vi "SM - Save settings to non-volatile memory.vi"(1 "error in":errorcluster, 2 "Address / Port":i16=1 min=1 max=31 step=1) -> (0 "error out":errorcluster)   [LabVIEW 2014]
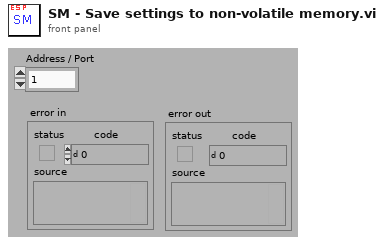
[diagram p1: front panel]
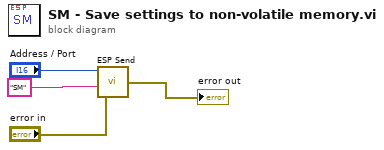
[diagram p0: block diagram]
diagram:
  n1 = call "ESP Send.vi"("Address / Port"="Address / Port", "Command String"="SM" ("Substring"), "error in"="error in") -> ("error out"=→"error out":errorcluster)  [unwired: 5 in]
